vi "AG33XXX.id query.vi"(0 "i ref in":refnum<vi>, 3 "ms timeout (10000)":i32=10000, 5 "error in (no error)":errorcluster) -> (14 "i ref out":refnum<vi>, 16 "IDString":string, 17 "timed out":bool, 19 "error out":errorcluster)   [LabVIEW 2014, in "AG33XXX.lvlib"]
doc: "Performs an ID query of the device."
uses:
  AG33XXX.lvlib
  CS_Core/CSApplicationBaseClasses/DeviceBase/DeviceBase.lvlib
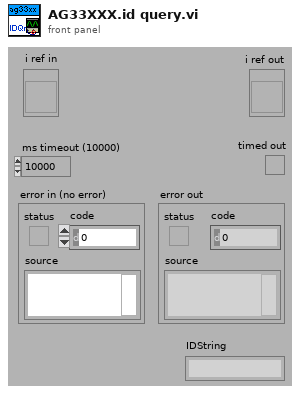
[diagram p1: front panel]
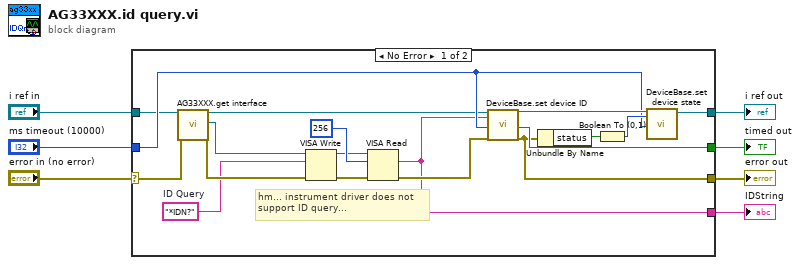
[diagram p0: block diagram]
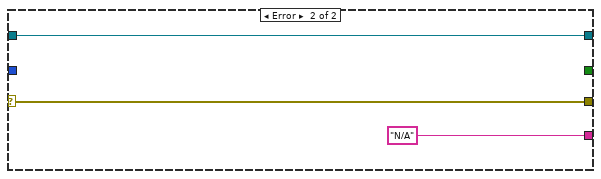
[diagram p2: hidden frame]
diagram:
  n1 = case shown="No Error" "error in (no error)" {
    selector: "error in (no error)" -> [w17 w27]
    tunnel: [w25 _] -> w7
    tunnel: [w20 w28] -> w6
    tunnel: "ms timeout (10000)" -> [w19 _]
    tunnel: "i ref in" -> [w18 w28]
    tunnel: [w21 w27] -> w2
    tunnel: [w13 "N/A"] -> w1
    frame No Error {
      w11 = "*IDN?"  # ID Query
      # "hm... instrument driver does not\nsupport ID query..."
      n2 = call "AG33XXX.get interface.vi"("i ref in"=w18, "error in (no error)"=w17) -> ("i ref out"=w12:refnum<vi>, "interface"=w16:refnum<visa-resource-name>, "error out"=w15:errorcluster)  [unwired: 15 in]
      n3 = VISA Write(VISA resource name=w16, write buffer=w11, error in (no error)=w15) -> (VISA resource name out=w8:refnum<visa-resource-name>, error out=w9:errorcluster)  [unwired: 1 out]
      n4 = VISA Read(VISA resource name=w8, byte count=u32 256, error in (no error)=w9) -> (read buffer=w13:string, error out=w14:errorcluster)  [unwired: 2 out]
      n5 = call "DeviceBase.set device ID.vi"("i ref in"=w12, "deviceID"=w13, "ms timeout (10000)"=w19, "error in (no error)"=w14) -> ("i ref out"=w22:refnum<vi>, "timed out"=w25:bool, "error out"=w21:errorcluster)  [unwired: 13 in]
      n6 = Unbundle By Name(w21) -> ("status"=w24:bool)
      n7 = Boolean To (0,1)(Boolean=w24) -> (0, 1=w23:i16)
      n8 = call "DeviceBase.set device state.vi"("i ref in"=w22, "deviceState"=w23, "ms timeout (10000)"=w19) -> ("i ref out"=w20:refnum<vi>)  [unwired: 14 in, 2 out]
    }
    frame Error {
    }
  }
  "error out" <- w2
  "i ref out" <- w6
  "timed out" <- w7
  "IDString" <- w1
